vi "Roller Arm Position.vi"(10 "Right Pot":dbl, 11 "Left Pot":dbl) -> (0 "Pot Diff":dbl, 1 "Right Closed?":bool, 2 "Left Closed?":bool, 3 "Portrait?":bool)   [LabVIEW 2014]
uses:
  Robot Global Data.vi
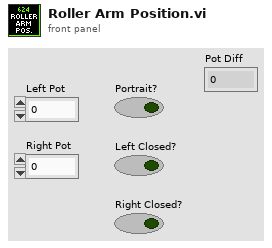
[diagram p1: front panel]
types:
  T1 = typedef "Dashboard Control Data.ctl" = cluster{"Cam Exposure":dbl, "Go to angle":dbl, "Steer PID Gains":cluster{"proportional gain (Kc)":dbl, "integral time (Ti, min)":dbl, "derivative time (Td, min)":dbl}, "Steer PID output Range":cluster{"output high":dbl, "output low":dbl}, "Pressure m \nValue":dbl, "Pressure b \nValue":dbl, "Strafe Timer\nWait":dbl, "Roller Command Cluster ":T2, "Elevator":T3, "Strafe Correct max steer":dbl, "IMU Enable":bool, "Encoder Control":T5, "IMU Controls":cluster{"Pitch Zero":dbl, "Roll Zero":dbl}}
  T2 = typedef "Roller Control.ctl" = cluster{"Intake Speed":dbl, "Turn In Speed":dbl, "Unload Speed":dbl, "Turn Out Speed":dbl, "Ping Align Tolerance":dbl, "Tote Range Threshold":dbl, "Right Pot 0":dbl, "Pot Threshold":dbl, "Left Pot 0":dbl, "Manual 0s?":bool, "Right Pot Scale":dbl, "Left Pot Scale":dbl, "0 wait time":i32, "Zero Pots":bool, "Min Elevator Height":dbl, "Eject Time":dbl, "Eject US Threshold":dbl, "Anti-Twitch Time":u32, "Ping Caring Threshold":dbl, "Pot Diff Threshold":dbl}
  T3 = typedef "Elevator DB Control.ctl" = cluster{"PID Output Range":cluster{"output high":dbl, "output low":dbl}, "PID gains":cluster{"proportional gain (Kc)":dbl, "integral time (Ti, min)":dbl, "derivative time (Td, min)":dbl}, "Height Tolerance":sgl, " Encoder Constant":dbl, "Safe Mode Max Speed":sgl, "Eject Time":sgl, "Zeroing Speed":sgl, "Presets":T4, "Ping Detect Threshold":sgl, "Trashcan Detect Threshold":sgl, "Zero Filter Time":dbl}
  T4 = typedef "Elevator Presets.ctl" = cluster{"Hold Tote":sgl, "Hold Trashcan":sgl, "Pickup 2 w/ Tote":sgl, "Pickup 2 w/ Trashcan":sgl, "Pickup 3 w/ Tote":sgl, "Pickup 3 w/ Trashcan":sgl, "Bottom":sgl, "Pickup 1 w/ Tote":sgl, "Pickup Trashcan":sgl, "Pickup 1 w/ Trashcan":sgl, "Eject":sgl, "Hold 6":sgl, "Step add height":sgl, "Store Trashcan 3":sgl, "Store Trashcan 4":sgl, "Store Trashcan 5":sgl, "6 Tote Max Height":sgl, "5 Tote Max Height":sgl}
  T5 = typedef "Encoder Control.ctl" = cluster{"Left Tick Constant":dbl, "Right Tick Constant":dbl, "Center Tick Constant":dbl, "Reset?":bool, "Y Dist":cluster{"PID gains":cluster{"proportional gain (Kc)":dbl, "integral time (Ti, min)":dbl, "derivative time (Td, min)":dbl}, "output range":cluster{"output high":dbl, "output low":dbl}}, "X Dist":cluster{"PID gains":cluster{"proportional gain (Kc)":dbl, "integral time (Ti, min)":dbl, "derivative time (Td, min)":dbl}, "output range":cluster{"output high":dbl, "output low":dbl}}, "Y Stop Thresh":dbl, "Y Stop Speed":dbl, "X Stop Thresh":dbl, "X Stop Speed":dbl}
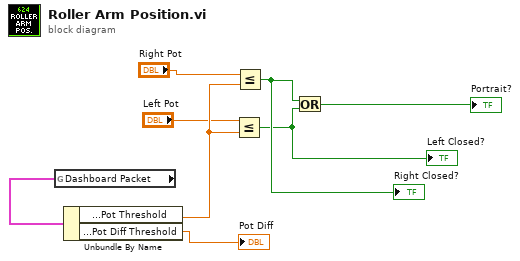
[diagram p0: block diagram]
diagram:
  n1 = global read "Robot Global Data.vi" "Dashboard Packet"() -> (w7:T1)
  n2 = Unbundle By Name(w7) -> ("Roller Command Cluster.Pot Threshold"=w8:dbl, "Roller Command Cluster.Pot Diff Threshold"=→"Pot Diff":dbl)
  n3 = Less Or Equal?(x="Left Pot", y=w8) -> (x <= y?=w3:bool)
  "Left Closed?" <- w3
  n4 = Less Or Equal?(x="Right Pot", y=w8) -> (x <= y?=w4:bool)
  "Right Closed?" <- w4
  n5 = Or(x=w4, y=w3) -> (x .or. y?=→"Portrait?":bool)
